vi "Object orientation + robot control with controlled grab.vi"() -> ()   [LabVIEW 2018]
uses:
  Underlying VI's/I2C Master VI/Arduino_Interfacing.ctl
  Underlying VI's/I2C Master VI/I2C_MASTER_WRITE_NEW Type Def.ctl
  Underlying VI's/NavX VI/navX type def.ctl
  <vilib>/userdefined/High Color/IMAQdx.ctl
  Underlying VI's/Modified webcam FGV/Webcam AE.ctl
  <vilib>/Studica/Studica Toolkit/Background/I2C Channel.ctl
  Underlying VI's/Motor Control VI with PID/MOTOR CONTROL WITH PID AE DATA MODE TYPE DEF.ctl
  Underlying VI's/Motor Control VI with PID/MOTOR CONTROL WITH PID AE DIRECTION TYPE DEF.ctl
  <vilib>/Studica/Studica Toolkit/NavX/NavX.lvlib
panel:
  in  "Mode 2":T1=enum."Read Values"
  in  "stop 2":bool
  out "NavX Readings":T2
  in  "Speed":dbl
  out "Corrected":dbl
  out "error":sgl
  out "error out":errorcluster
  in  "Data to Write":T3
  in  "AE Mode":T4
  in  "Grab":bool
  in  "ENA":bool
  out "Error out":errorcluster
  in  "stop":bool
  out "Image":T5(plugin-control)
  out "Object Center Coordinates":cluster{"x":sgl, "y":sgl}
  out "Object detection cluster":T6
  in  "Mode":enum16{"Ball", "Soap", "Gel", "Pipe", "None"}(ring)
  # "Save me pls"
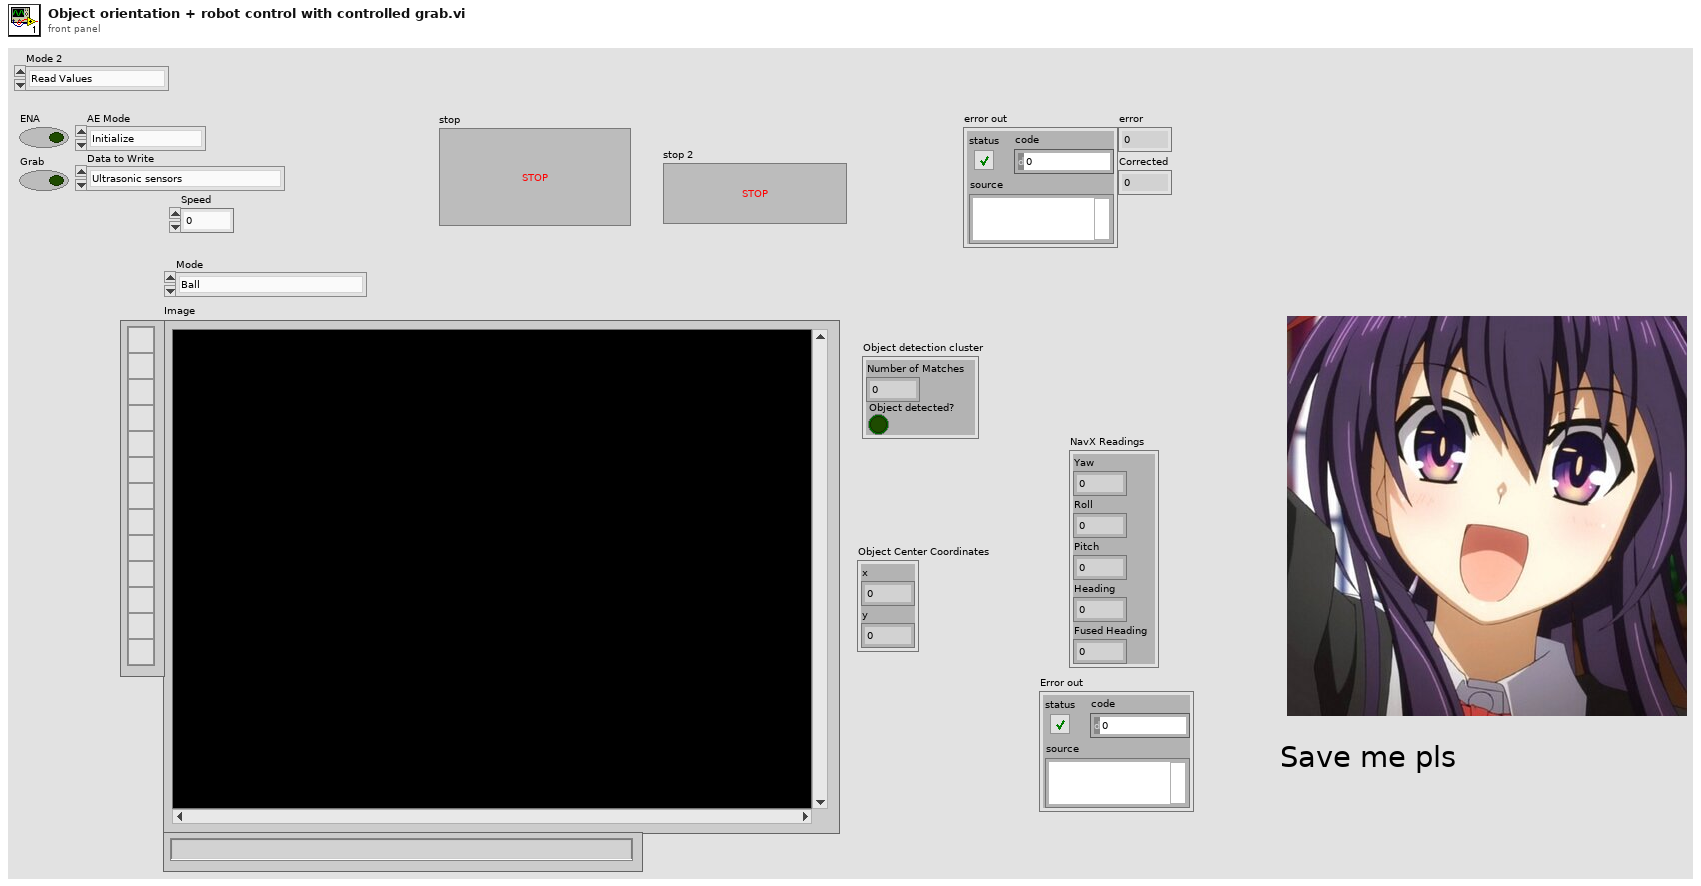
[diagram p1: front panel]
types:
  T1 = typedef "navX type def.ctl" = enum16{"Get i2C reference", "Read Values", "Zero Yaw"}
  T2 = cluster{"Yaw":dbl, "Roll":dbl, "Pitch":dbl, "Heading":dbl, "Fused Heading":dbl}
  T3 = typedef "I2C_MASTER_WRITE_NEW Type Def.ctl" = enum16{"Ultrasonic sensors", "Stepper origin", "zStepper 13.3k", "zStepper 13k", "zStepper 12k", "zStepper 11k", "zStepper 10k", "zStepper 9k", "zStepper 8k", "zStepper 7k", "zStepper 6k", "zStepper 5k", "zStepper 4k", "zStepper 3k", "zStepper 2k", "zStepper 1k", "zStepper 900", "zStepper 800", "zStepper 700", "zStepper 600", "zStepper 500", "zStepper 400", "zStepper 300", "zStepper 200", "zStepper 100", "zStepper 0", "yStepper control", "Open Claw", "Close Claw", "Soft Reset"}
  T4 = typedef "Arduino_Interfacing.ctl" = enum16{"Initialize", "Write to Arduino", "Read From Arduino"}
  T5 = typedef "IMAQ Image.ctl" = refnum<image>
  T6 = cluster{"Number of Matches":i32, "Object detected?":bool}
  T7 = typedef "Webcam AE.ctl" = enum16{"Initialize Camera", "Open Camera", "Continuous Acquisition", "Close Camera", "Retrieve Image", "Dispose Camera Image Buffer"}
  T8 = typedef "IMAQdx.ctl" = refnum<k21>
  T9 = typedef "I2C Channel.ctl" = enum16{"Not Connected", "A", "B"}
  T10 = cluster{"I2C Ref Out":cluster{"I2C Channel":T9, "FPGA VI Reference Out":refnum<k20>}, "Connected":bool, "Slave Address (7-bit)":u8, "Registry":u8[]}
  T11 = typedef "MOTOR CONTROL WITH PID AE DIRECTION TYPE DEF.ctl" = enum16{"y-axis movement", "x-axis movement", "rotation", "stop", "reset encoders"}
  T12 = typedef "MOTOR CONTROL WITH PID AE DATA MODE TYPE DEF.ctl" = enum16{"Init AE", "Write to AE", "Read from AE"}
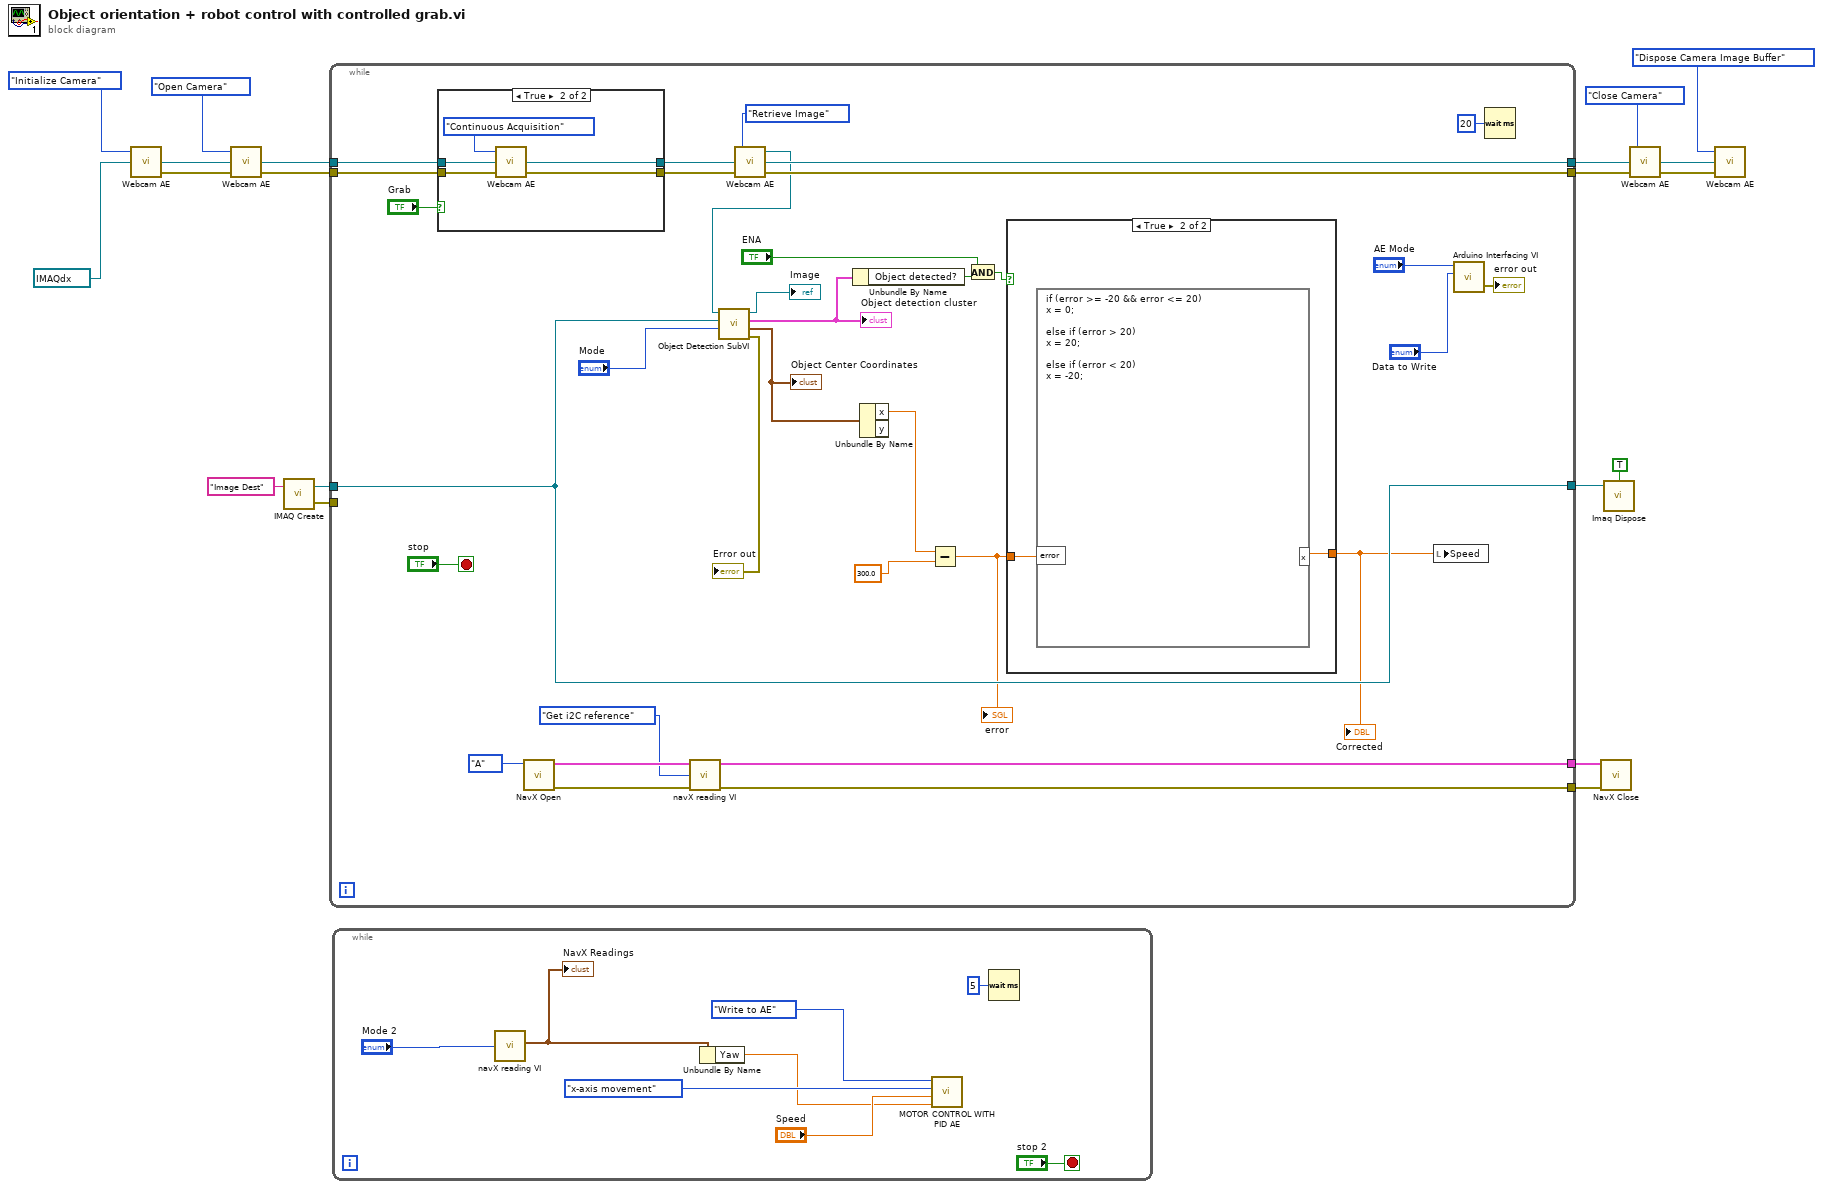
[diagram p0: block diagram]
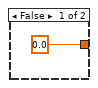
[diagram p3: hidden frame]
diagram:
  n1 = call "Webcam AE.vi"("Session In"=T8 "cam0", "Camera states"=Webcam_AE."Initialize Camera") -> ("error out"=w15:errorcluster, "Session Out"=w11:T8)  [unwired: 1 in, 1 out]
  n2 = call "Webcam AE.vi"("error in (no error)"=w15, "Session In"=w11, "Camera states"=Webcam_AE."Open Camera") -> ("error out"=w14:errorcluster, "Session Out"=w10:T8)  [unwired: 1 out]
  n3 = call "IMAQ Create"("Image Name"="Image Dest") -> ("New Image"=w20:T5, "error out"=w17:errorcluster)  [unwired: 4 in]
  n4 = while {
    tunnel: w20 -> [w49]
    tunnel: [w49] -> w18
    tunnel: w17 -> [_]
    tunnel: w14 -> [w42]
    tunnel: [w40] -> w13
    tunnel: w10 -> [w39]
    tunnel: [w37] -> w9
    tunnel: [w26] -> w1
    tunnel: [w25] -> w2
    stop <- "stop" stop-if-true
    n5 = case shown="True" "Grab" {
      tunnel: w42 -> [w54 w60]
      tunnel: [w54 w59] -> w41
      tunnel: w39 -> [w55 w58]
      tunnel: [w55 w57] -> w38
      frame False {
      }
      frame True {
        n6 = call "Webcam AE.vi"("error in (no error)"=w60, "Session In"=w58, "Camera states"=Webcam_AE."Continuous Acquisition") -> ("error out"=w59:errorcluster, "Session Out"=w57:T8)  [unwired: 1 out]
      }
    }
    n7 = call <vilib>:"NavX Open.vi"("I2C Channel"=I2C_Channel."A") -> ("error out"=w27:errorcluster, "NavX Info"=w29:T10)  [unwired: 9 in]
    n8 = call "navX reading VI.vi"("NavX Info In"=w29, "Mode"=navX_type_def."Get i2C reference" ("Mode 2"), "error in (no error)"=w27) -> ("NavX Info Out"=w26:T10, "Error Out"=w25:errorcluster)  [unwired: 2 out]
    n9 = call "Webcam AE.vi"("error in (no error)"=w41, "Session In"=w38, "Camera states"=Webcam_AE."Retrieve Image") -> ("error out"=w40:errorcluster, "Session Out"=w37:T8, "Image Out"=w34:T5)
    n10 = call "Object Detection SubVI.vi"("Mode"="Mode", "Image Dest"=w49, "Image in"=w34) -> ("Error out"=→"Error out":errorcluster, "Object Center Coordinates"=w47:cluster{"x":sgl, "y":sgl}, "Object detection cluster"=w46:T6, "Image Out"=→"Image":T5)  [unwired: 1 in]
    "Object detection cluster" <- w46
    "Object Center Coordinates" <- w47
    n11 = Unbundle By Name(w46) -> ("Object detected?"=w45:bool)
    n12 = Unbundle By Name(w47) -> ("x"=w33:sgl)  [unwired: 1 out]
    n13 = Subtract(x=w33, y=sgl 300.0) -> (x-y=w31:sgl)
    "error" <- w31
    n14 = And(x="ENA", y=w45) -> (x .and. y?=w43:bool)
    n15 = case shown="True" w43 {
      tunnel: [0.0 ("y") w62] -> w21
      tunnel: w31 -> [_ w63]
      frame False {
      }
      frame True {
        n16 = formula code="if (error >= -20 && error <= 20)\nx = 0;\n\nelse if (error > 20)\nx = 20;\n\nelse if (error < 20)\nx = -20;"("error"=w63) -> ("x"=w62:dbl)
      }
    }
    "Corrected" <- w21
    n17 = local write "Speed"(w21) -> ()
    n18 = call "Arduino Interfacing VI.vi"("Data to Write"="Data to Write", "AE Mode"="AE Mode") -> ("error out"=→"error out":errorcluster)  [unwired: 2 in, 1 out]
    n19 = Wait (ms)(milliseconds to wait=u32 20) -> ()  [unwired: 1 out]
  }
  n20 = while {
    stop <- "stop 2" stop-if-true
    n21 = call "navX reading VI.vi"("Mode"="Mode 2") -> ("NavX Readings"=w66:T2)  [unwired: 2 in, 3 out]
    "NavX Readings" <- w66
    n22 = Unbundle By Name(w66) -> ("Yaw"=w65:dbl)
    n23 = call "MOTOR CONTROL WITH PID AE.vi"("Yaw"=w65, "Speed"="Speed", "Direction"=MOTOR_CONTROL_WITH_PID_AE_DIRECTION_TYPE_DEF."x-axis movement", "AE Mode"=MOTOR_CONTROL_WITH_PID_AE_DATA_MODE_TYPE_DEF."Write to AE") -> ()  [unwired: 1 out]
    n24 = Wait (ms)(milliseconds to wait=u32 5) -> ()  [unwired: 1 out]
  }
  n25 = call <vilib>:"NavX Close.vi"("error in (no error)"=w2, "NavX Info In"=w1) -> ()  [unwired: 9 in, 1 out]
  n26 = call "Imaq Dispose"("All Images? (No)"=TRUE, "Image"=w18) -> ()  [unwired: 4 in, 1 out]
  n27 = call "Webcam AE.vi"("error in (no error)"=w13, "Session In"=w9, "Camera states"=Webcam_AE."Close Camera") -> ("error out"=w12:errorcluster, "Session Out"=w8:T8)  [unwired: 1 out]
  n28 = call "Webcam AE.vi"("error in (no error)"=w12, "Session In"=w8, "Camera states"=Webcam_AE."Dispose Camera Image Buffer") -> ()  [unwired: 3 out]
